vi "Ensure Discovery Service Started.vi"(8 "error in (no error)":errorcluster, 11 "Path":path) -> (0 "error out":errorcluster, 3 "Key File Path":path)   [LabVIEW 2020, in "MeasurementLink Measurement Server.lvlib"]
uses:
  MeasurementLink Measurement Server.lvlib
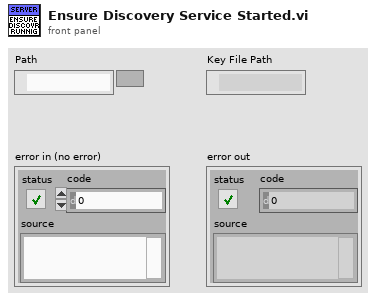
[diagram p1: front panel]
types:
  T1 = enum16{"open", "replace", "create", "open or create", "replace or create", "replace or create with confirmation"}
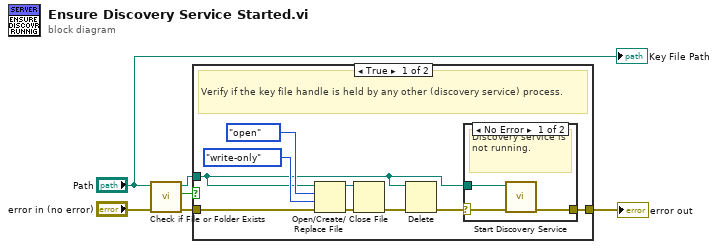
[diagram p0: block diagram]
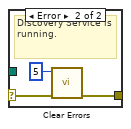
[diagram p2: hidden frame]
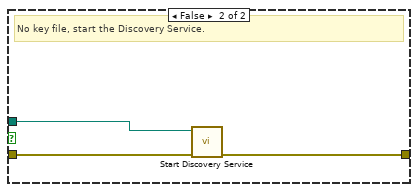
[diagram p3: hidden frame]
diagram:
  n1 = call <vilib>:"Check if File or Folder Exists.vi"("error in (no error)"="error in (no error)", "path"="Path") -> ("error out"=w6:errorcluster, "file or folder exists?"=w5:bool, "dup path"=w2:path)  [unwired: 7 in]
  n2 = case shown="True" w5 {
    tunnel: w6 -> [w12 w24]
    tunnel: [w13 w23] -> w3
    tunnel: w2 -> [w7 w22]
    frame True {
      # "Verify if the key file handle is held by any other (discovery service) process."
      n3 = Open/Create/Replace File(file path (use dialog)=w7, error in=w12, operation (0:open)=T1."open", access (0:read/write)=enum16{"read/write", "read-only", "write-only"}."write-only") -> (refnum out=w9:refnum<file>, error out=w10:errorcluster)  [unwired: 2 in, 1 out]
      n4 = Close File(refnum=w9, error in=w10) -> (error out=w8:errorcluster)  [unwired: 1 out]
      n5 = Delete(path (use dialog)=w7, error in=w8) -> (error out=w11:errorcluster)  [unwired: 3 in, 2 out]
      n6 = case shown="No Error" w11 {
        selector: w11 -> [w18 w21]
        tunnel: [w17 w20] -> w13
        tunnel: w7 -> [w16 _]
        frame No Error {
          # "Discovery service is not running."
          n7 = call "Start Discovery Service.vi"("error in"=w18, "Key File Path"=w16) -> ("error out"=w17:errorcluster)  [unwired: 9 in]
        }
        frame Error {
          # "Discovery Service is running."
          n8 = call <vilib>:"Clear Errors.vi"("error in (no error)"=w21, "specific error code to clear (0: all)"=5) -> ("error out"=w20:errorcluster)  [unwired: 4 in, 1 out]
        }
      }
    }
    frame False {
      # "No key file, start the Discovery Service."
      n9 = call "Start Discovery Service.vi"("error in"=w24, "Key File Path"=w22) -> ("error out"=w23:errorcluster)  [unwired: 9 in]
    }
  }
  "error out" <- w3
  "Key File Path" <- "Path"
